vi "Insert SubPanel.vi"(8 "error in (no error)":errorcluster, 10 "VI Ref":refnum<vi>, 11 "Subpanel Ref":refnum<vi>) -> (0 "error out":errorcluster)   [LabVIEW 2020]
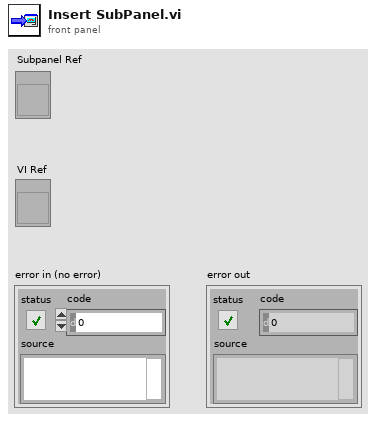
[diagram p1: front panel]
types:
  T1 = enum32{"Invalid", "Standard", "Closed", "Hidden", "Minimized", "Maximized"}
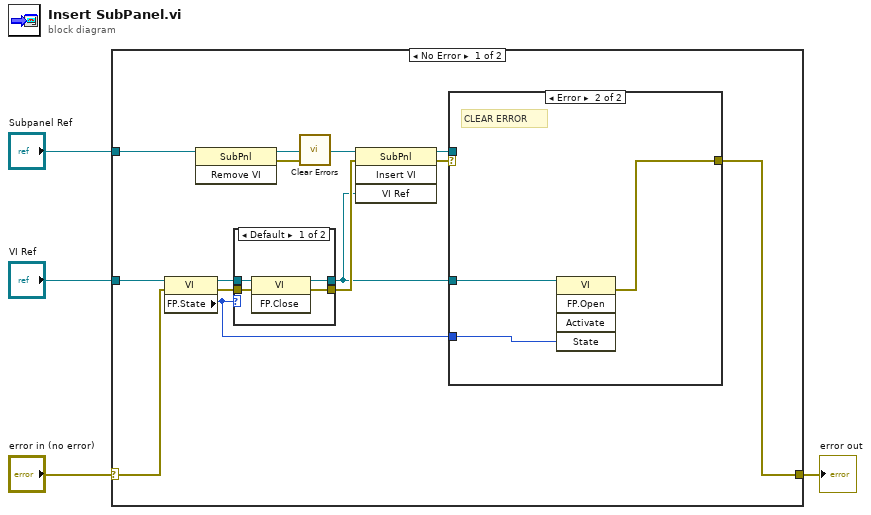
[diagram p0: block diagram]
diagram:
  n1 = case shown="No Error" "error in (no error)" {
    selector: "error in (no error)" -> [w9 w28]
    tunnel: "VI Ref" -> [w17 _]
    tunnel: "Subpanel Ref" -> [w7 _]
    tunnel: [w8 w28] -> w1
    frame No Error {
      n2 = property class="VI"(reference=w17, error in=w9) -> (reference out=w16:refnum<vi>, error out=w15:errorcluster, "FP.State"=w10:T1)
      n3 = invoke class="SubPnl" method="Remove VI"(reference=w7) -> (reference out=w6:refnum<vi>, error out=w5:errorcluster)  [unwired: 2 in, 1 out]
      n4 = case shown="Default" w10 {
        tunnel: w16 -> [w21 w23]
        tunnel: w15 -> [w20 w22]
        tunnel: [w19 w23] -> w11
        tunnel: [w18 w22] -> w14
        frame Default {
          n5 = invoke class="VI" method="FP.Close"(reference=w21, error in=w20) -> (reference out=w19:refnum<vi>, error out=w18:errorcluster)  [unwired: 1 in, 1 out]
        }
        frame "Closed" {
        }
      }
      n6 = call <vilib>:"Clear Errors.vi"("error in (no error)"=w5) -> ()  [unwired: 5 in, 2 out]
      n7 = invoke class="SubPnl" method="Insert VI"(reference=w6, error in=w14, "VI Ref"=w11) -> (reference out=w12:refnum<vi>, error out=w13:errorcluster)  [unwired: 1 in, 2 out]
      n8 = case shown="Error" w13 {
        selector: w13 -> [w24 _]
        tunnel: w12 -> [_ _]
        tunnel: w11 -> [_ w27]
        tunnel: w10 -> [_ w26]
        tunnel: [w24 w25] -> w8
        frame No Error {
        }
        frame Error {
          # "CLEAR ERROR"
          n9 = invoke class="VI" method="FP.Open"(reference=w27, "State"=w26) -> (error out=w25:errorcluster)  [unwired: 3 in, 4 out]
        }
      }
    }
    frame Error {
    }
  }
  "error out" <- w1
